vi "WPI_UtilitiesFRCAutomaticValuePublisher.vi"() -> ()   [LabVIEW 2025]
panel:
  in  "Enable":bool=TRUE
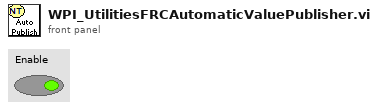
[diagram p1: front panel]
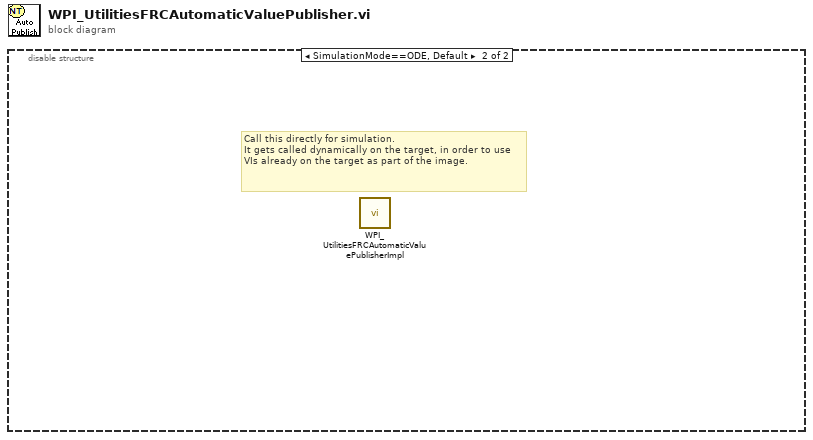
[diagram p0: block diagram]
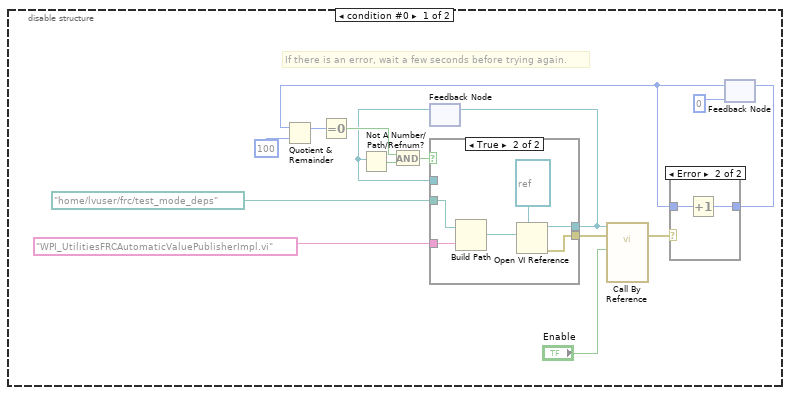
[diagram p2: hidden frame]
diagram:
  n1 = disable-structure shown="SimulationMode==ODE, Default" {
    frame condition #0 {
      # "If there is an error, wait a few seconds before trying again."
      n2 = feedback #1() -> (w4:refnum<vi>)  [unwired: 1 in]
      n3 = Not A Number/Path/Refnum?(number/path/refnum=w4) -> (NaN/Path/Refnum?=w13:bool)
      n4 = feedback #2(0) -> (w15:i32)
      n5 = Quotient & Remainder(x=w15, y=100) -> (x-y*floor(x/y)=w11:i32)  [unwired: 1 out]
      n6 = Equal To 0?(x=w11) -> (x = 0?=w12:bool)
      n7 = And(x=w12, y=w13) -> (x .and. y?=w14:bool)
      n8 = case shown="True" w14 {
        tunnel: [w19 w24] -> w3
        tunnel: w4 -> [w19 _]
        tunnel: "WPI_UtilitiesFRCAutomaticValuePublisherImpl.vi" -> [_ w22]
        tunnel: path "/home/lvuser/frc/test_mode_deps" -> [_ w21]
        tunnel: [_ w20] -> w6
        frame False {
        }
        frame True {
          n9 = Build Path(base path=w21, name or relative path=w22) -> (appended path=w23:path)
          n10 = Open VI Reference(type specifier VI Refnum (for type only)=refnum<vi> refnum, vi path=w23) -> (vi reference=w24:refnum<vi>, error out=w20:errorcluster)  [unwired: 4 in]
        }
      }
      n11 = feedback-in #1(w3) -> ()
      n12 = call-by-ref "?"(reference=w3, error in=w6, "Enable"="Enable") -> (error out=w7:errorcluster)  [unwired: 11 in, 1 out]
      n13 = case shown="Error" w7 {
        tunnel: [w16 w18] -> w8
        tunnel: w15 -> [w16 w17]
        frame No Error {
        }
        frame Error {
          n14 = Increment(x=w17) -> (x+1=w18:i32)
        }
      }
      n15 = feedback-in #2(w8) -> ()
    }
    frame condition #1 (active) {
      # "Call this directly for simulation.\nIt gets called dynamically on the target, in order to use VIs already on the target as part of the image."
      n16 = call <vilib>:"WPI_UtilitiesFRCAutomaticValuePublisherImpl.vi"() -> ()  [unwired: 12 in]
    }
  }
